vi "reql_table_list.vi"(6 "ms timeout (0:default)":i32, 7 "db name":string, 8 "error in (no error)":errorcluster, 11 "rethinkdb in":refnum<class "RethinkDB.lvclass">) -> (0 "error out":errorcluster, 2 "table list":string[](array[string]), 3 "rethinkdb out":refnum<class "RethinkDB.lvclass">, 4 "response":variant)   [LabVIEW 2017, in "rethinkdb.lvlib"]
uses:
  rethinkdb.lvlib
  RethinkDB.lvclass
  ql2_term.ctl
  ql2_query.ctl
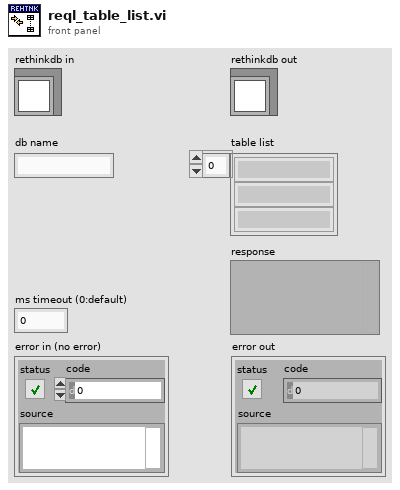
[diagram p1: front panel]
types:
  T1 = typedef "rethinkdb.lvlib/ql2_query.ctl" = enum8{"START", "CONTINUE", "STOP", "NOREPLY_WAIT", "SERVER_INFO", "invalid"}
  T2 = typedef "rethinkdb.lvlib/ql2_term.ctl" = enum8{"ADD", "AND", "APPEND", "APRIL", "ARGS", "ASC", "AUGUST", "AVG", "BETWEEN", "BETWEEN_DEPRECATED", "BINARY", "BIT_AND", "BIT_NOT", "BIT_OR", "BIT_SAL", "BIT_SAR", "BIT_XOR", "BRACKET", "BRANCH", "CEIL", "CHANGES", "CHANGE_AT", "CIRCLE", "COERCE_TO", "CONCAT_MAP", "CONFIG", "CONTAINS", "COUNT", "DATE", "DATUM", "DAY", "DAY_OF_WEEK", "DAY_OF_YEAR", "DB", "DB_CREATE", "DB_DROP", "DB_LIST", "DECEMBER", "DEFAULT", "DELETE", "DELETE_AT", "DESC", "DIFFERENCE", "DISTANCE", "DISTINCT", "DIV", "DOWNCASE", "DURING", "EPOCH_TIME", "EQ", "EQ_JOIN", "ERROR", "FEBRUARY", "FILL", "FILTER", "FLOOR", "FOLD", "FOR_EACH", "FRIDAY", "FUNC", "FUNCALL", "GE", "GEOJSON", "GET", "GET_ALL", "GET_FIELD", "GET_INTERSECTING", "GET_NEAREST", "GET_WRITE_HOOK", "GRANT", "GROUP", "GT", "HAS_FIELDS", "HOURS", "HTTP", "IMPLICIT_VAR", "INCLUDES", "INDEX_CREATE", "INDEX_DROP", "INDEX_LIST", "INDEX_RENAME", "INDEX_STATUS", "INDEX_WAIT", "INFO", "INNER_JOIN", "INSERT", "INSERT_AT", "INTERSECTS", "IN_TIMEZONE", "ISO8601", "IS_EMPTY", "JANUARY", "JAVASCRIPT", "JSON", "JULY", "JUNE", "KEYS", "LE", "LIMIT", "LINE", "LITERAL", "LT", "MAKE_ARRAY", "MAKE_OBJ", "MAP", "MARCH", "MATCH", "MAX", "MAXVAL", "MAY", "MERGE", "MIN", "MINUTES", "MINVAL", "MOD", "MONDAY", "MONTH", "MUL", "NE", "NOT", "NOVEMBER", "NOW", "NTH", "OBJECT", "OCTOBER", "OFFSETS_OF", "OR", "ORDER_BY", "OUTER_JOIN", "PLUCK", "POINT", "POLYGON", "POLYGON_SUB", "PREPEND", "RANDOM", "RANGE", "REBALANCE", "RECONFIGURE", "REDUCE", "REPLACE", "ROUND", "SAMPLE", "SATURDAY", "SECONDS", "SEPTEMBER", "SET_DIFFERENCE", "SET_INSERT", "SET_INTERSECTION", "SET_UNION", "SET_WRITE_HOOK", "SKIP", "SLICE", "SPLICE_AT", "SPLIT", "STATUS", "SUB", "SUM", "SUNDAY", "SYNC", "TABLE", "TABLE_CREATE", "TABLE_DROP", "TABLE_LIST", "THURSDAY", "TIME", "TIMEZONE", "TIME_OF_DAY", "TO_EPOCH_TIME", "TO_GEOJSON", "TO_ISO8601", "TO_JSON_STRING", "TUESDAY", "TYPE_OF", "UNGROUP", "UNION", "UPCASE", "UPDATE", "UUID", "VALUES", "VAR", "WAIT", "WEDNESDAY", "WITHOUT", "WITH_FIELDS", "YEAR", "ZIP", "invalid"}
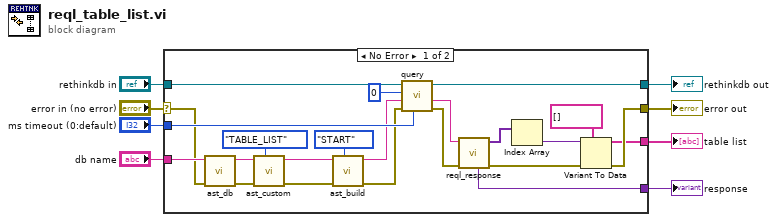
[diagram p0: block diagram]
diagram:
  n1 = case shown="No Error" "error in (no error)" {
    selector: "error in (no error)" -> [w11 w33]
    tunnel: "rethinkdb in" -> [w31 w32]
    tunnel: [w30 w32] -> w6
    tunnel: "ms timeout (0:default)" -> [w29 _]
    tunnel: [w23 w33] -> w4
    tunnel: [w20 _] -> w3
    tunnel: "db name" -> [w14 _]
    tunnel: [w19 _] -> w1
    frame No Error {
      n2 = call "ast_db.vi"("error in (no error)"=w11, "db name"=w14) -> ("error out"=w18:errorcluster, "r.db"=w15:string)  [unwired: 8 in]
      n3 = call "ast_custom.vi"("term_type"=ql2_term."TABLE_LIST", "error in (no error)"=w18, "arg0"=w15) -> ("error out"=w17:errorcluster, "r"=w16:string)  [unwired: 7 in]
      n4 = call "ast_build.vi"("query_type"=ql2_query."START", "error in (no error)"=w17, "term"=w16) -> ("error out"=w9:errorcluster, "query"=w10:string)  [unwired: 7 in]
      n5 = call "query.vi"("ms timeout (0:default)"=w29, "error in (no error)"=w9, "query"=w10, "token in (random)"=u64 0, "rethinkdb in"=w31) -> ("error out"=w27:errorcluster, "response"=w25:string, "rethinkdb out"=w30:refnum<class "RethinkDB.lvclass">)  [unwired: 3 in, 1 out]
      n6 = call "reql_response.vi"("error in (no error)"=w27, "response"=w25) -> ("error out"=w26:errorcluster, "values"=w24:variant[], "response"=w19:variant)  [unwired: 7 in]
      n7 = Index Array(array=w24) -> (element=w22:variant)  [unwired: 1 in]
      n8 = Variant To Data(error in=w26, type=string[] [], Variant=w22) -> (data=w20:string[], error out=w23:errorcluster)
    }
    frame Error {
    }
  }
  "error out" <- w4
  "rethinkdb out" <- w6
  "table list" <- w3
  "response" <- w1
